vi "notifyObserver.vi"(8 "error in (no error)":errorcluster, 11 "WeatherData.lvclass":refnum<class "WeatherData.lvclass">) -> (0 "error out":errorcluster, 3 "WeatherData.lvclass 2":refnum<class "WeatherData.lvclass">)   [LabVIEW 2020, in "WeatherData.lvclass"]
uses:
  WeatherData.lvclass
  WeatherData.lvclass/WeatherData.ctl
  Observer/Observer.lvclass
panel:
  # "Connector Pane"
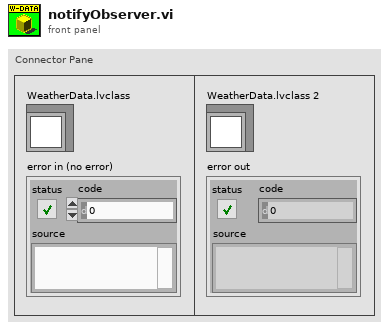
[diagram p1: front panel]
types:
  T1 = typedef "weatherDataCluster.ctl" = cluster{"Temperature":dbl, "Humidity":dbl, "Pressure":dbl, "Observers":refnum<class "Observer.lvclass">[]}
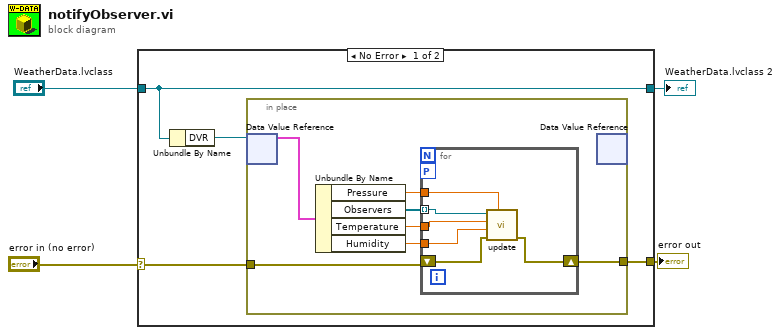
[diagram p0: block diagram]
diagram:
  n1 = case shown="No Error" "error in (no error)" {
    selector: "error in (no error)" -> [w8 w22]
    tunnel: [w7 w22] -> w3
    tunnel: "WeatherData.lvclass" -> [w5 w23]
    tunnel: [w5 w23] -> w1
    frame No Error {
      n2 = Unbundle By Name(w5) -> ("DVR"=w6:refnum<data-value>)
      n3 = in-place {
        in-place-border: w8 -> [w11]
        in-place-border: [w10] -> w7
        n4 = in-place-dvr #1(w6) -> (w9:T1)  [unwired: 1 out]
        n5 = Unbundle By Name(w9) -> ("Pressure"=w14:dbl, "Observers"=w15:refnum<class "Observer.lvclass">[], "Temperature"=w13:dbl, "Humidity"=w12:dbl)
        n6 = for {
          tunnel: w15 -> [w21] mode=indexing
          tunnel: w14 -> [w20]
          tunnel: w13 -> [w19]
          tunnel: w12 -> [w18]
          shift-right: [w16] -> w10
          shift-left: w11 -> [w17]
          workers-P: _ -> [_]
          n7 = call-dynamic "update.vi"("Pressure"=w20, "error in (no error)"=w17, "Humidity"=w18, "Temperature"=w19, "Observer.lvclass"=w21) -> ("error out"=w16:errorcluster)  [unwired: 5 in, 1 out]
        }
        n8 = in-place-dvr #1() -> ()  [unwired: 1 in, 2 out]
      }
    }
    frame Error {
    }
  }
  "error out" <- w3
  "WeatherData.lvclass 2" <- w1
